vi "ErrorLog_GetAllErrors.vi"(8 "error in (no error)":errorcluster, 11 "reference in":refnum<class "ErrorLog.lvclass">) -> (0 "error out":errorcluster, 1 "Errors since last call":string, 2 "New Errors":bool, 3 "reference out":refnum<class "ErrorLog.lvclass">, 4 "Errors since last clear":string, 5 "Uncleared Errors":bool, 6 "Error owners since last clear":string[](array[string]), 7 "Error owners since last call":string[](array[string]))   [LabVIEW 2023, in "ErrorLog.lvclass"]
uses:
  ErrorLog.lvclass
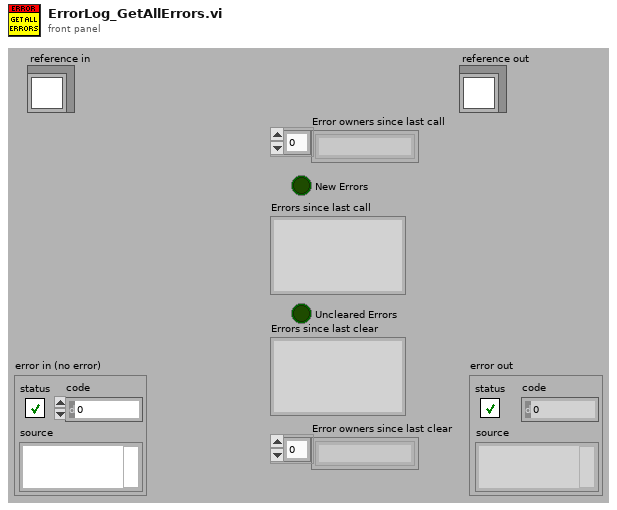
[diagram p1: front panel]
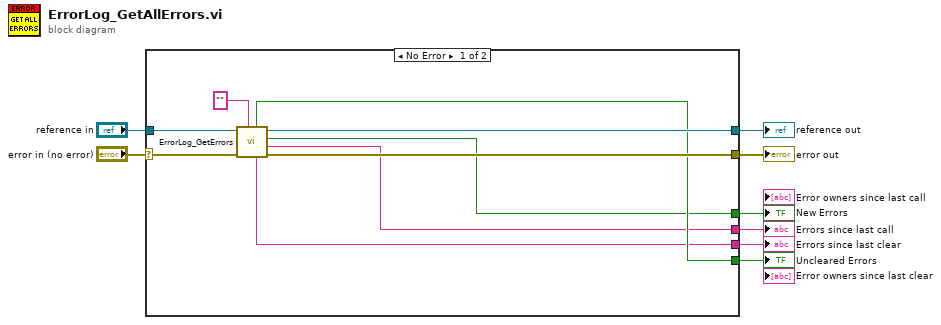
[diagram p0: block diagram]
diagram:
  n1 = case shown="No Error" "error in (no error)" {
    selector: "error in (no error)" -> [w16 w19]
    tunnel: [w15 w19] -> w7
    tunnel: [w14 w18] -> w5
    tunnel: "reference in" -> [w17 w18]
    tunnel: [w11 _] -> w4
    tunnel: [w10 _] -> w3
    tunnel: [w12 _] -> w2
    tunnel: [w13 _] -> w1
    frame No Error {
      n2 = call-dynamic "ErrorLog_GetErrors.vi"("Owner"="", "error in (no error)"=w16, "reference in"=w17) -> ("error out"=w15:errorcluster, "Errors since last call"=w11:string, "New Errors"=w12:bool, "reference out"=w14:refnum<class "ErrorLog.lvclass">, "Errors since last clear"=w10:string, "Uncleared Errors"=w13:bool)  [unwired: 3 in]
    }
    frame Error {
    }
  }
  "error out" <- w7
  "reference out" <- w5
  "Errors since last call" <- w4
  "New Errors" <- w2
  "Errors since last clear" <- w3
  "Uncleared Errors" <- w1
